vi "emi_VI Recursive Self call.vi"() -> (8 "Recursive Self Call?":bool)   [LabVIEW 2011]
doc: "Returns true if the VI called it self.\n\nUsed to seperate first call, from self call in recursive VIs\n\nsubrouting reentrant for efficiensy\n\nError tunnels skipped from lack of need, and speed"
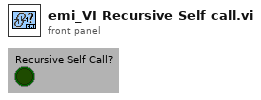
[diagram p1: front panel]
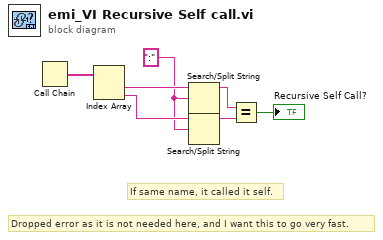
[diagram p0: block diagram]
diagram:
  w4 = ":" ("search string/char (-)")
  # "If same name, it called it self."
  # "Dropped error as it is not needed here, and I want this to go very fast."
  n1 = Call Chain() -> (call chain=w7:string[])
  n2 = Index Array(array=w7) -> (element #1=w6:string, element #2=w5:string)  [unwired: 2 in]
  n3 = Search/Split String(string=w6, search string/char (-)=w4) -> (substring before match=w2:string)  [unwired: 1 in, 2 out]
  n4 = Search/Split String(string=w5, search string/char (-)=w4) -> (substring before match=w3:string)  [unwired: 1 in, 2 out]
  n5 = Equal?(x=w2, y=w3) -> (x = y?=→"Recursive Self Call?":bool)
